vi "Test Find Tests With Amp Sign.vi"(8 "error in (no error)":errorcluster, 11 "Test Case In":refnum<class "Test FInder Test.lvclass">) -> (0 "error out":errorcluster, 3 "Test Case Out":refnum<class "Test FInder Test.lvclass">)   [LabVIEW 2020, in "Test FInder Test.lvclass"]
uses:
  Test FInder Test.lvclass
  Test FInder Test.lvclass/Test FInder Test.ctl
  source/Framework/Test Finder/Test Finder.lvclass
  source/LUnit Test Suite.lvclass
  1012ae70-2596-402a-939d-7405f7103d79.vi
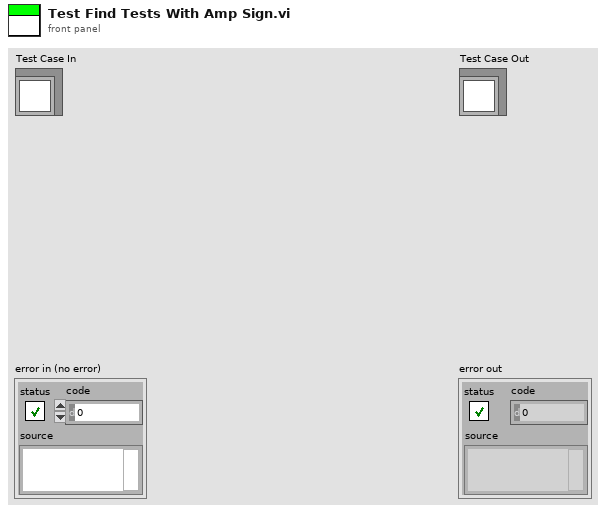
[diagram p1: front panel]
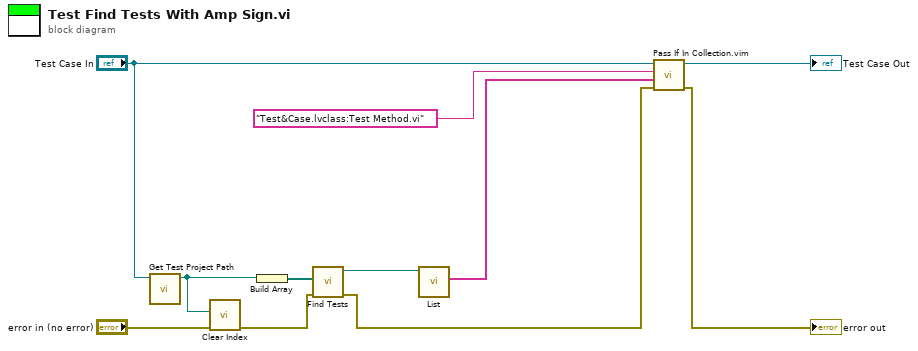
[diagram p0: block diagram]
diagram:
  n1 = call "Get Test Project Path.vi"("LUnit Test Suite Tests in"="Test Case In") -> ("appended path"=w3:path)  [unwired: 10 in]
  n2 = call "Clear Index.vi"("error in (no error)"="error in (no error)", "Project Path"=w3) -> ("error out"=w4:errorcluster)  [unwired: 9 in]
  n3 = Build Array(w3) -> (w8:path[])
  n4 = call "Find Tests.vi"("error in (no error)"=w4, "File Paths"=w8) -> ("error out"=w9:errorcluster, "LUnit Test Suite"=w7:refnum<class "LUnit Test Suite.lvclass">)  [unwired: 8 in]
  n5 = call "List.vi"("LUnit Test Suite In"=w7) -> ("List of Runnables"=w2:string[])  [unwired: 9 in, 1 out]
  n6 = call "Pass If In Collection.vim"("error in (no error)"=w9, "Collection"=w2, "Expected Element"="Test&Case.lvclass:Test Method.vi", "LUnit Test Case In"="Test Case In") -> ("error out"=→"error out":errorcluster, "LUnit Test Case Out"=→"Test Case Out":refnum<class "Test FInder Test.lvclass">)  [unwired: 6 in]
